vi "A.vi"(8 "A error in (no error)":errorcluster, 11 "Numeric":dbl) -> (0 "error out":errorcluster)   [LabVIEW 2017]
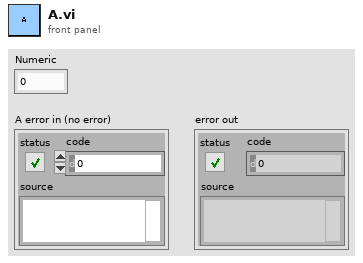
[diagram p1: front panel]
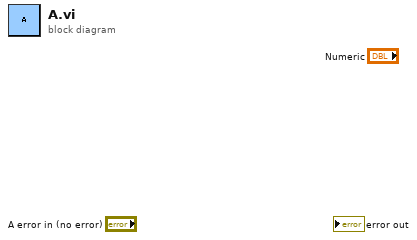
[diagram p0: block diagram]
diagram:
